vi "FSK 2bits.vi"() -> ()   [LabVIEW 2010]
panel:
  out "Tableau 2":bool[](array[boolean])
  out "Graphe déroulant":dynamicdata(graph)
  in  "Tableau":bool[](array[boolean])
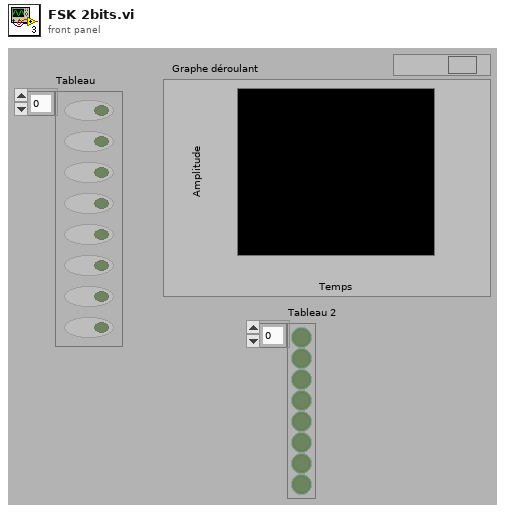
[diagram p1: front panel]
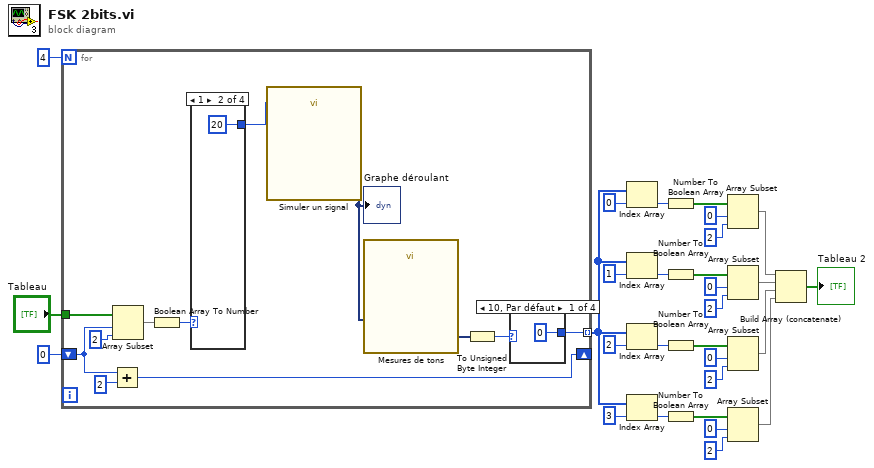
[diagram p0: block diagram]
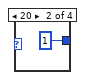
[diagram p2: hidden frame]
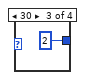
[diagram p3: hidden frame]
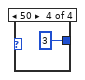
[diagram p4: hidden frame]
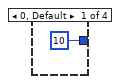
[diagram p5: hidden frame]
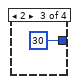
[diagram p6: hidden frame]
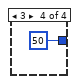
[diagram p7: hidden frame]
diagram:
  n1 = for {
    N: 4 -> [_]
    shift-right: [w40] -> _
    shift-left: 0 -> [w39]
    tunnel: "Tableau" -> [w37]
    tunnel: [w33] -> w22 mode=indexing
    n2 = Add(x=w39, y=2) -> (x+y=w40:i32)
    n3 = Array Subset(array=w37, index=w39, length=2) -> (w36:bool[])
    n4 = Boolean Array To Number(Boolean array=w36) -> (number=w34:u32)
    n5 = case shown="1" w34 {
      tunnel: [10 20 30 50] -> w31
      frame 0, Default {
      }
      frame 1 {
      }
      frame 2 {
      }
      frame 3 {
      }
    }
    n6 = call "Simuler un signal"("Frequency"=w31) -> ("Sinus"=w35:dynamicdata)  [unwired: 13 in, 1 out]
    "Graphe déroulant" <- w35
    n7 = call "Mesures de tons"("Signals"=w35) -> ("Frequency"=w30:dynamicdata)  [unwired: 9 in, 1 out]
    n8 = To Unsigned Byte Integer(number=w30) -> (unsigned 8bit integer=w32:u8)
    n9 = case shown="10, Par défaut" w32 {
      tunnel: [0 1 2 3] -> w33
      frame 10, Default {
      }
      frame 20 {
      }
      frame 30 {
      }
      frame 50 {
      }
    }
  }
  n10 = Index Array(array=w22, index=0) -> (element=w7:i32)
  n11 = Index Array(array=w22, index=1) -> (element=w9:i32)
  n12 = Index Array(array=w22, index=2) -> (element=w12:i32)
  n13 = Index Array(array=w22, index=3) -> (element=w13:i32)
  n14 = Number To Boolean Array(number=w7) -> (Boolean array=w6:bool[])
  n15 = Number To Boolean Array(number=w9) -> (Boolean array=w8:bool[])
  n16 = Number To Boolean Array(number=w12) -> (Boolean array=w11:bool[])
  n17 = Number To Boolean Array(number=w13) -> (Boolean array=w10:bool[])
  n18 = Array Subset(array=w6, index=0, length=2) -> (w5:bool[])
  n19 = Array Subset(array=w8, index=0, length=2) -> (w4:bool[])
  n20 = Array Subset(array=w11, index=0, length=2) -> (w3:bool[])
  n21 = Array Subset(array=w10, index=0, length=2) -> (w2:bool[])
  n22 = Build Array (concatenate)(w5, w4, w3, w2) -> (→"Tableau 2":bool[])
